vi "Ctor.vi"(8 "error in (no error)":errorcluster, 11 "Websocket Server in":refnum<class "Websocket Server.lvclass">) -> (0 "error out":errorcluster, 3 "Websocket Server out":refnum<class "Websocket Server.lvclass">)   [LabVIEW 2020, in "Stream-Websocket.lvlib" / "Websocket Server.lvclass"]
uses:
  Websocket Server.lvclass
  Websocket Client/Websocket Client.lvclass
  Ref Data.ctl
  Listener Status.ctl
  Stream-Websocket.lvlib
  Listener Result.ctl
  lv-stream/stream/Endpoint/Endpoint.lvclass
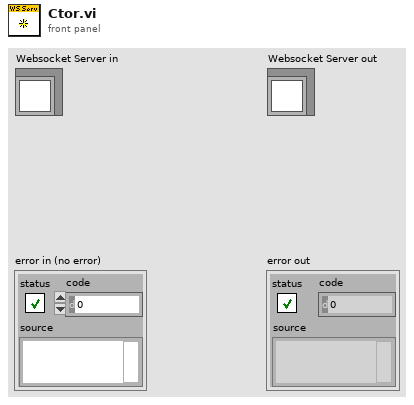
[diagram p1: front panel]
types:
  T1 = typedef "Stream-Websocket.lvlib/Listener Result.ctl" = cluster{"Status":T2, "Client":refnum<class "Websocket Client.lvclass">}
  T2 = typedef "Stream-Websocket.lvlib/Listener Status.ctl" = enum16{"Successful", "Unsuccessful"}
  T3 = typedef "Stream-Websocket.lvlib/Websocket Server.lvclass/Ref Data.ctl" = cluster{"Listener":refnum<k5>, "Clients":refnum<class "Websocket Client.lvclass">[], "Open":bool}
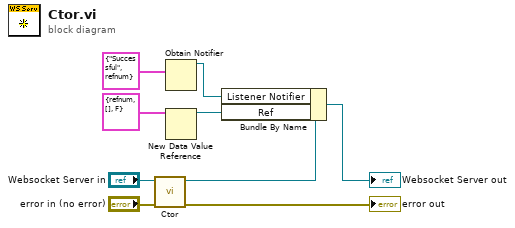
[diagram p0: block diagram]
diagram:
  n1 = call-parent "Ctor.vi"("error in (no error)"="error in (no error)", "Endpoint in"="Websocket Server in") -> ("error out"=→"error out":errorcluster, "Endpoint out"=w6:refnum<class "Websocket Server.lvclass">)  [unwired: 8 in]
  n2 = Obtain Notifier(notification data type=T1 {"Status"=enum."Successful", "Client"=refnum} ("Listener Result")) -> (notifier out=w1:refnum<notifier>)  [unwired: 3 in, 2 out]
  n3 = New Data Value Reference(data value=T3 {"Listener"=refnum, "Clients"=[], "Open"=FALSE} ("Ref Data")) -> (data value reference=w4:refnum<data-value>)  [unwired: 1 in, 1 out]
  n4 = Bundle By Name(cluster=w6, "Listener Notifier"=w1, "Ref"=w4) -> (→"Websocket Server out":refnum<class "Websocket Server.lvclass">)
